vi "1DStandardConteniousPlot_LPF.vi"() -> ()   [LabVIEW 2024]
uses:
  <vilib>/DAQmx/read.llb/DAQmx Read (Analog 1D DBL 1Chan NSamp).vi
  <vilib>/DAQmx/create/channels.llb/DAQmx Create Channel (AI-Voltage-Basic).vi
  <vilib>/DAQmx/configure/timing.llb/DAQmx Timing (Sample Clock).vi
  <vilib>/DAQmx/miscellaneous.llb/DAQmx Fill In Error Info.vi
panel:
  in  "Lower Cut-Off":dbl=5.0
  out "Waveform Graph":dynamicdata(graph)
  in  "stop":bool
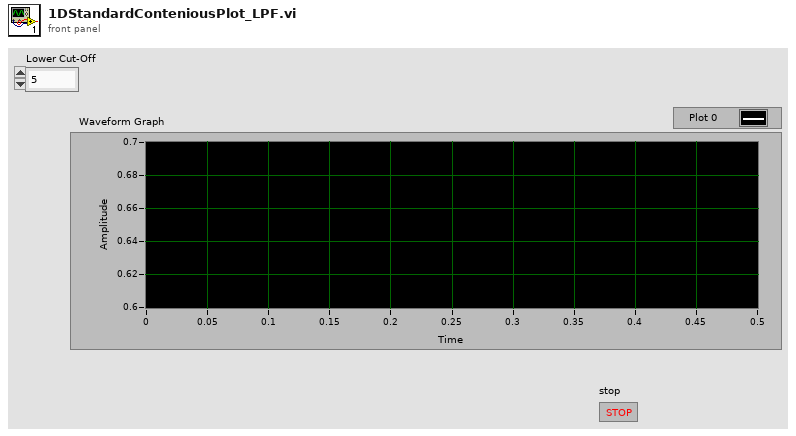
[diagram p1: front panel]
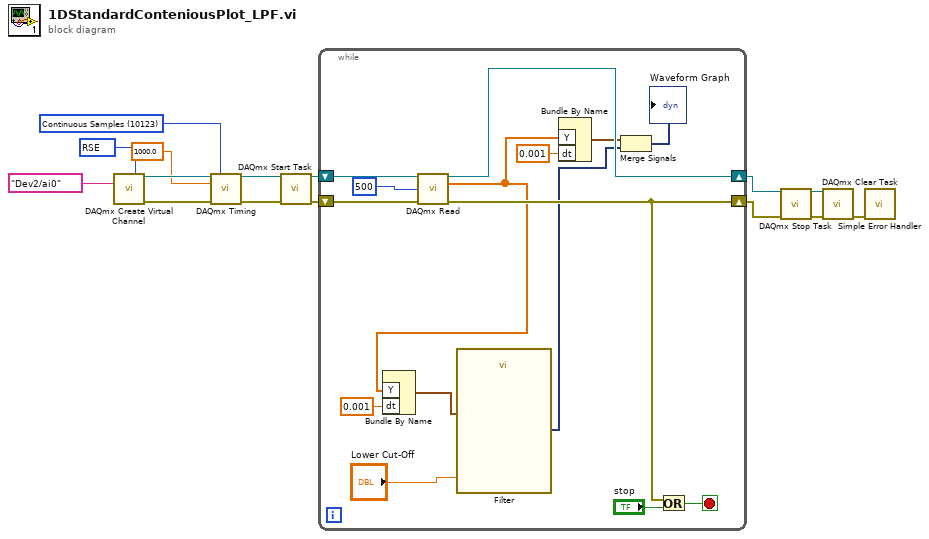
[diagram p0: block diagram]
diagram:
  w1 = 10083 items=["Default"=-1, "RSE"=10083, "NRSE"=10078, "Differential"=10106, "Pseudodifferential"=12529] ("input terminal configuration")
  w11 = 10123 items=["Finite Samples"=10178, "Continuous Samples"=10123, "Hardware Timed Single Point"=12522] ("sample mode")
  n1 = call-poly <vilib>:"DAQmx Create Virtual Channel.vi"("input terminal configuration"=w1, "physical channels"=tag "Dev2/ai0") -> ("task out"=w14:refnum<k21>, "error out"=w13:errorcluster)  [unwired: 12 in]
  n2 = call-poly <vilib>:"DAQmx Timing.vi"("task/channels in"=w14, "sample mode"=w11, "rate"=1000.0, "error in"=w13) -> ("task out"=w10:refnum<k21>, "error out"=w9:errorcluster)  [unwired: 10 in]
  n3 = call <vilib>:"DAQmx Start Task.vi"("task/channels in"=w10, "error in"=w9) -> ("task out"=w8:refnum<k21>, "error out"=w7:errorcluster)  [unwired: 12 in]
  n4 = while {
    shift-right: [w27] -> w6
    shift-left: w8 -> [w30]
    shift-right: [w25] -> w5
    shift-left: w7 -> [w29]
    stop <- w24 stop-if-true
    n5 = call-poly <vilib>:"DAQmx Read.vi"("task/channels in"=w30, "number of samples per channel"=500, "error in"=w29) -> ("task out"=w27:refnum<k21>, "data"=w20:dbl[], "error out"=w25:errorcluster)  [unwired: 10 in]
    n6 = Bundle By Name("Y"=w20, "dt"=0.001) -> (w21:waveform(dbl))  [unwired: 1 in]
    n7 = call "Filter"("Lower Cut-Off"="Lower Cut-Off", "Signal"=w21) -> ("Filtered Signal"=w16:dynamicdata)  [unwired: 8 in, 1 out]
    n8 = Bundle By Name("Y"=w20, "dt"=0.001) -> (w18:waveform(dbl))  [unwired: 1 in]
    n9 = Merge Signals(w18, w16) -> (→"Waveform Graph":dynamicdata)
    n10 = Or(x=w25, y="stop") -> (x .or. y?=w24:bool)
  }
  n11 = call <vilib>:"DAQmx Stop Task.vi"("task/channels in"=w6, "error in"=w5) -> ("task out"=w4:refnum<k21>, "error out"=w3:errorcluster)  [unwired: 12 in]
  n12 = call <vilib>:"DAQmx Clear Task.vi"("task in"=w4, "error in"=w3) -> ("error out"=w2:errorcluster)  [unwired: 13 in]
  n13 = call <vilib>:"Simple Error Handler.vi"("error in (no error)"=w2) -> ()  [unwired: 4 in, 5 out]
